vi "square.vi"(8 "error in (no error)":errorcluster, 11 "params":refnum<class "JSON Value.lvclass">) -> (0 "error out":errorcluster, 3 "data":refnum<class "JSON Value.lvclass">)   [LabVIEW 2017]
uses:
  <vilib>/NI/JSON Support for LabVIEW/JSON Value/JSON Value.lvclass
  <vilib>/NI/JSON Support for LabVIEW/JSON Types.ctl
  <vilib>/NI/JSON Support for LabVIEW/JSON Value/Read Value/Read value (Numeric).vi
  <vilib>/NI/JSON Support for LabVIEW/JSON Value/New JSON Value/New JSON (Numeric).vi
panel:
  out "datatype":T1
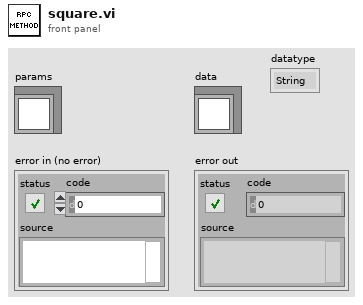
[diagram p1: front panel]
types:
  T1 = typedef "JSON Value.lvclass/JSON Types.ctl" = enum16{"String", "Numeric", "Boolean", "NULL", "Object", "Array"}
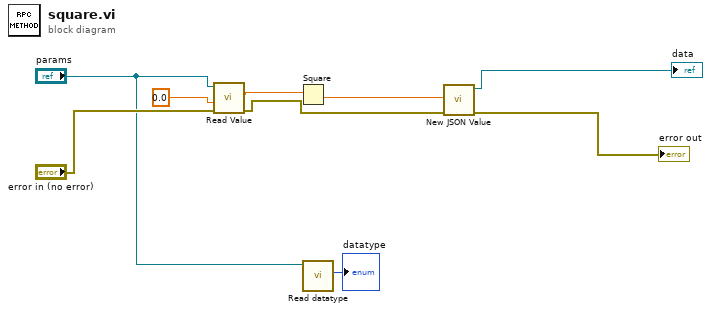
[diagram p0: block diagram]
diagram:
  n1 = call-poly <vilib>:"Read Value.vi"("error in (no error)"="error in (no error)", "default value"=0.0, "JSON Numeric in"="params") -> ("error out"=w3:errorcluster, "value"=w4:dbl)  [unwired: 6 in, 1 out]
  n2 = Square(x=w4) -> (x^2=w9:dbl)
  n3 = call <vilib>:"Read datatype.vi"("JSON Value in"="params") -> ("datatype"=→"datatype":T1)  [unwired: 8 in, 2 out]
  n4 = call-poly <vilib>:"New JSON Value.vi"("error in (no error)"=w3, "value"=w9) -> ("error out"=→"error out":errorcluster, "JSON Value out"=→"data":refnum<class "JSON Value.lvclass">)  [unwired: 8 in]
